vi "Search 1D String Array All Matches.vi"(2 "Element":string, 3 "1D String Array":string[](array[string])) -> (0 "Index[]":i32[](array[numeric]))   [LabVIEW 2014, in "SLL String.lvlib"]
doc: "Search 1D String Array for a specified element ignoring white space and case sensitivity"
uses:
  SLL String.lvlib
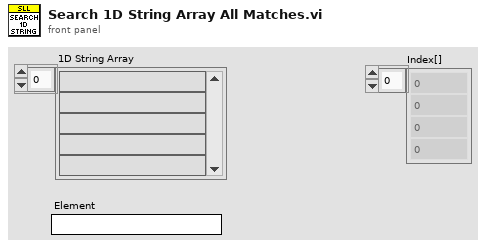
[diagram p1: front panel]
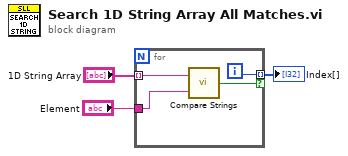
[diagram p0: block diagram]
diagram:
  n1 = for {
    tunnel: "1D String Array" -> [w7] mode=indexing
    tunnel: "Element" -> [w6]
    tunnel: [w5] -> w1 mode=indexing if=w4
    i -> [w5]
    n2 = call "Compare Strings.vi"("y"=w6, "x"=w7) -> ("Equal?"=w4:bool)
  }
  "Index[]" <- w1
